vi "sum Array.vi"() -> ()   [LabVIEW 2023]
panel:
  out "Numeric":dbl
  out "Numeric 2":dbl
  in  "array 2":dbl[](array[numeric])
  in  "array":dbl[](array[numeric])
  # "For loop"
  # "While loop"
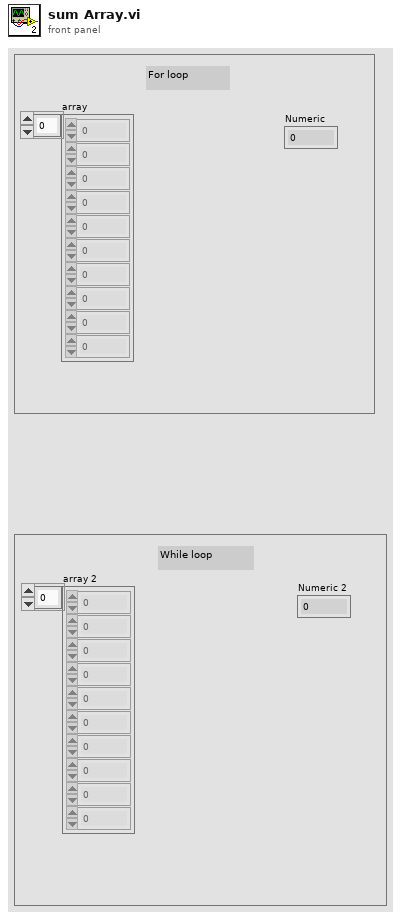
[diagram p1: front panel]
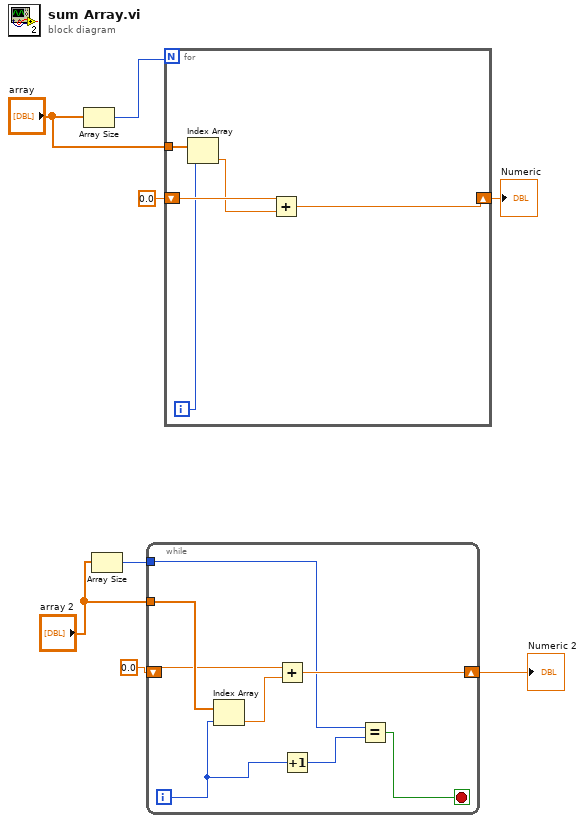
[diagram p0: block diagram]
diagram:
  n1 = Array Size(array="array") -> (size(s)=w8:i32)
  n2 = Array Size(array="array 2") -> (size(s)=w5:i32)
  n3 = while {
    tunnel: w5 -> [w12]
    tunnel: "array 2" -> [w16]
    shift-right: [w14] -> w3
    shift-left: 0.0 -> [w9]
    i -> [w13]
    stop <- w10 stop-if-true
    n4 = Index Array(array=w16, index=w13) -> (element=w15:dbl)
    n5 = Add(x=w9, y=w15) -> (x+y=w14:dbl)
    n6 = Increment(x=w13) -> (x+1=w11:i32)
    n7 = Equal?(x=w12, y=w11) -> (x = y?=w10:bool)
  }
  "Numeric 2" <- w3
  n8 = for {
    N: w8 -> [_]
    shift-right: [w20] -> w1
    shift-left: 0.0 -> [w21]
    tunnel: "array" -> [w19]
    i -> [w18]
    n9 = Index Array(array=w19, index=w18) -> (element=w17:dbl)
    n10 = Add(x=w21, y=w17) -> (x+y=w20:dbl)
  }
  "Numeric" <- w1
